vi "add.vi"(8 "error in (no error)":errorcluster, 11 "params":refnum<class "JSON Value.lvclass">) -> (0 "error out":errorcluster, 3 "data":refnum<class "JSON Value.lvclass">)   [LabVIEW 2017]
uses:
  <vilib>/NI/JSON Support for LabVIEW/JSON Value/JSON Value.lvclass
  <vilib>/NI/JSON Support for LabVIEW/JSON Value/Array/Index Array/Index Array (Numeric).vi
  <vilib>/NI/JSON Support for LabVIEW/JSON Value/New JSON Value/New JSON (Numeric).vi
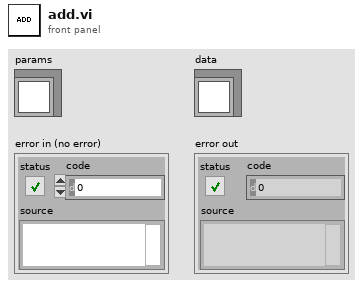
[diagram p1: front panel]
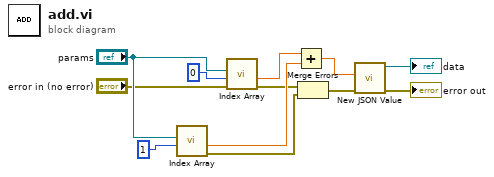
[diagram p0: block diagram]
diagram:
  n1 = call-poly <vilib>:"Index Array.vi"("index"=1, "JSON Value in"="params") -> ("error out"=w4:errorcluster, "Numeric"=w8:dbl)  [unwired: 8 in]
  n2 = call-poly <vilib>:"Index Array.vi"("error in (no error)"="error in (no error)", "index"=0, "JSON Value in"="params") -> ("error out"=w5:errorcluster, "Numeric"=w9:dbl)  [unwired: 7 in]
  n3 = Add(x=w9, y=w8) -> (x+y=w7:dbl)
  n4 = Merge Errors(w5, w4) -> (w3:errorcluster)
  n5 = call-poly <vilib>:"New JSON Value.vi"("error in (no error)"=w3, "value"=w7) -> ("error out"=→"error out":errorcluster, "JSON Value out"=→"data":refnum<class "JSON Value.lvclass">)  [unwired: 8 in]
